vi "CCD3000 Pixel to Wavelength v10.1.0.vi"(2 "Wavelengths (nm)":dbl[](array[numeric]), 3 "Raw Spectrum":dbl[](array[numeric])) -> (0 "Spectrum-Array":dbl[][](array[numeric]), 1 "Spectrum-Cluster":T1(array[cluster]))   [LabVIEW 2010]
panel:
  out "Ausgangs-Cluster":T2
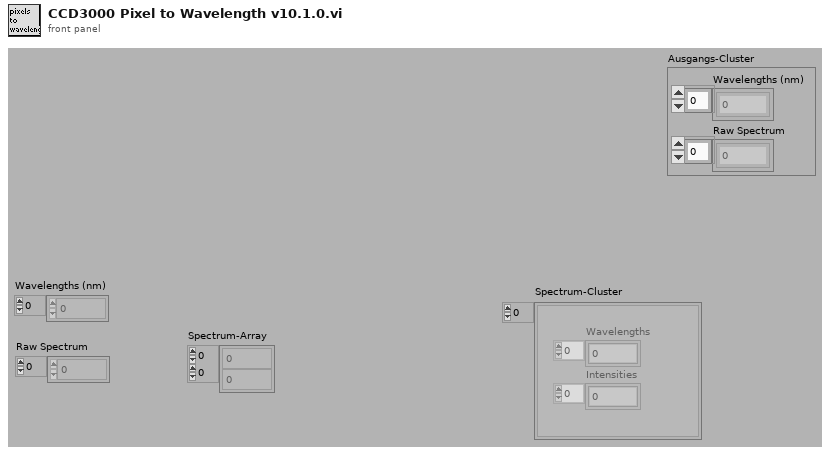
[diagram p1: front panel]
types:
  T1 = cluster{"Intensities":dbl[], "Wavelengths":dbl[]}[]
  T2 = cluster{"Wavelengths (nm)":dbl[], "Raw Spectrum":dbl[]}
  T3 = cluster{"Wavelengths (nm)":dbl[], "Raw Spectrum":dbl[]}[]
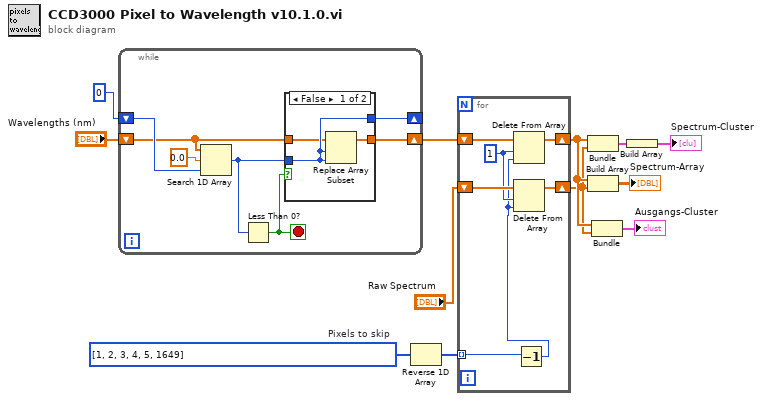
[diagram p0: block diagram]
diagram:
  w12 = i32[] [1, 2, 3, 4, 5, 1649]  # Pixels to skip
  n1 = while {
    shift-right: [w13] -> w8
    shift-left: "Wavelengths (nm)" -> [w16]
    shift-right: [w17] -> _
    shift-left: 0 ("index of element") -> [w18]
    stop <- w15 stop-if-true
    n2 = Search 1D Array(1D array=w16, element=0.0, start index (0)=w18) -> (index of element=w14:i32)
    n3 = Less Than 0?(x=w14) -> (x < 0?=w15:bool)
    n4 = case shown="False" w15 {
      tunnel: w14 -> [w22 w24]
      tunnel: [w22 w24] -> w17
      tunnel: w16 -> [w21 w23]
      tunnel: [w20 w23] -> w13
      frame False {
        n5 = Replace Array Subset(array=w21, new element=w22, index=w22) -> (w20:dbl[])
      }
      frame True {
      }
    }
  }
  n6 = Reverse 1D Array(array=w12) -> (reversed array=w6:i32[])
  n7 = for {
    shift-right: [w30] -> w5
    shift-left: w8 -> [w29]
    shift-right: [w31] -> w4
    shift-left: "Raw Spectrum" -> [w28]
    tunnel: w6 -> [w26] mode=indexing
    w27 = 1 ("length")
    n8 = Decrement(x=w26) -> (x-1=w25:i32)
    n9 = Delete From Array(array=w29, length=w27, index=w25) -> (array with subset deleted=w30:dbl[])  [unwired: 1 out]
    n10 = Delete From Array(array=w28, length=w27, index=w25) -> (array with subset deleted=w31:dbl[])  [unwired: 1 out]
  }
  n11 = Bundle("Wavelengths (nm)"=w5, "Raw Spectrum"=w4) -> (w2:T2)  [unwired: 1 in]
  n12 = Build Array(w5, w4) -> (→"Spectrum-Array":dbl[][])
  n13 = Bundle("Wavelengths (nm)"=w5, "Raw Spectrum"=w4) -> (→"Ausgangs-Cluster":T2)  [unwired: 1 in]
  n14 = Build Array(w2) -> (→"Spectrum-Cluster":T3)
